vi "IntakeCmdCancelALWAYS.vi"   [LabVIEW 2023]
uses:
  <vilib>/Rock Robotics/WPI/ThirdParty/JAS_Junk/TrajLib/VI/DigSeqLogic_Edge_On.vi
  <vilib>/Rock Robotics/WPI/ThirdParty/JAS_Junk/TrajLib/VI/BoolCmd_Send_Internal.vi
  <vilib>/Rock Robotics/WPI/ThirdParty/JAS_Junk/TrajLib/VI/BoolCmd_ObtainQueue.vi
  <vilib>/Rock Robotics/WPI/ThirdParty/JAS_Junk/TrajLib/Trajectory_Library.lvlib
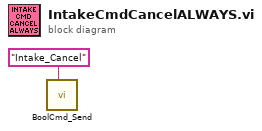
[diagram p0: block diagram]
diagram:
  n1 = call <vilib>:"BoolCmd_Send.vi"("Command Name"="Intake_Cancel") -> ()  [unwired: 10 in, 1 out]
